vi "MapDeviceErrorToDescription.vi"(8 "error in":errorcluster {"code" format="%.0x"}, 11 "device error":u16 format="%.0x") -> (0 "error out":errorcluster {"code" format="%.0x"}, 3 "element":string)   [LabVIEW 2016]
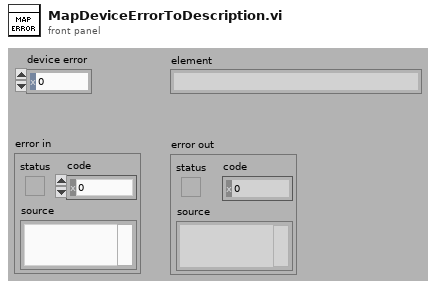
[diagram p1: front panel]
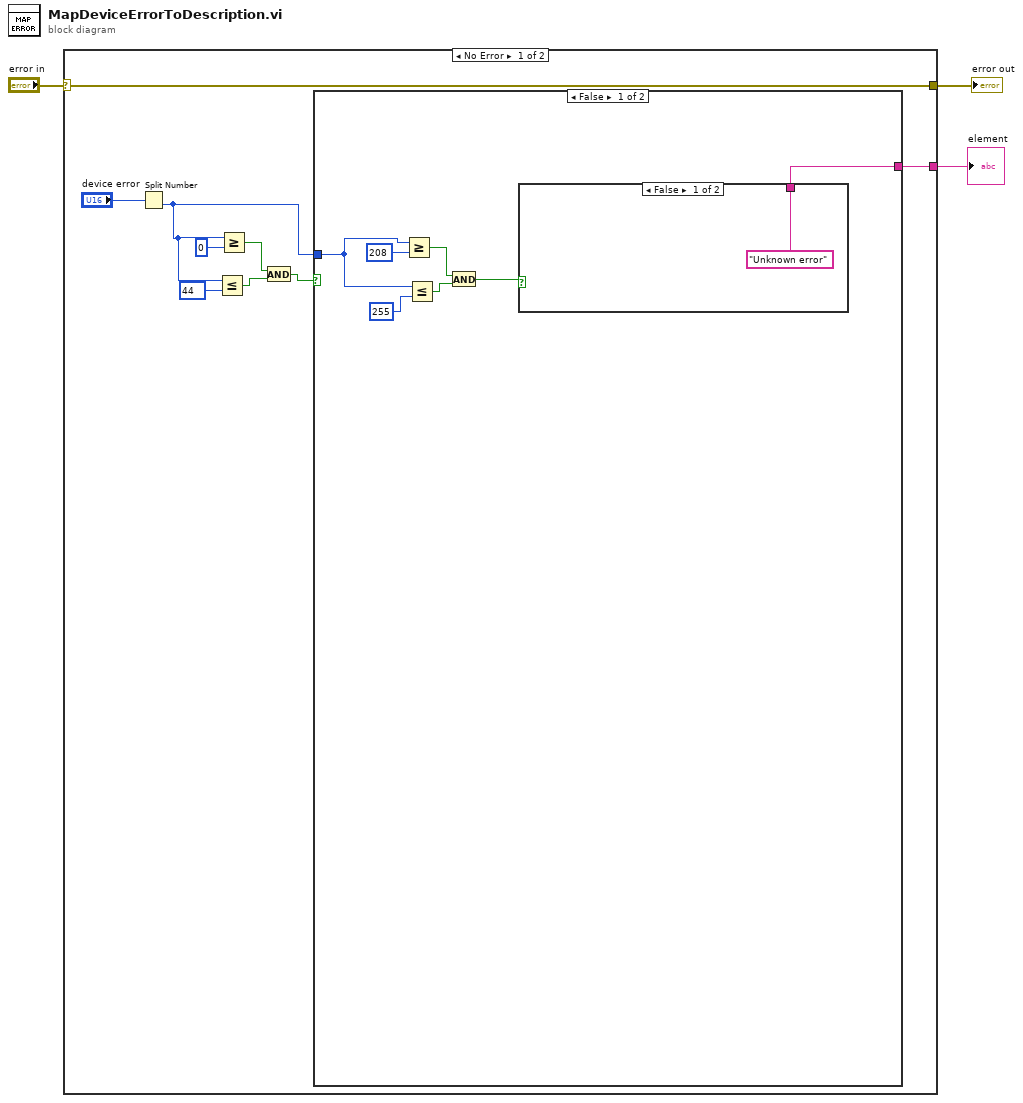
[diagram p0: block diagram]
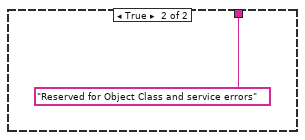
[diagram p2: hidden frame]
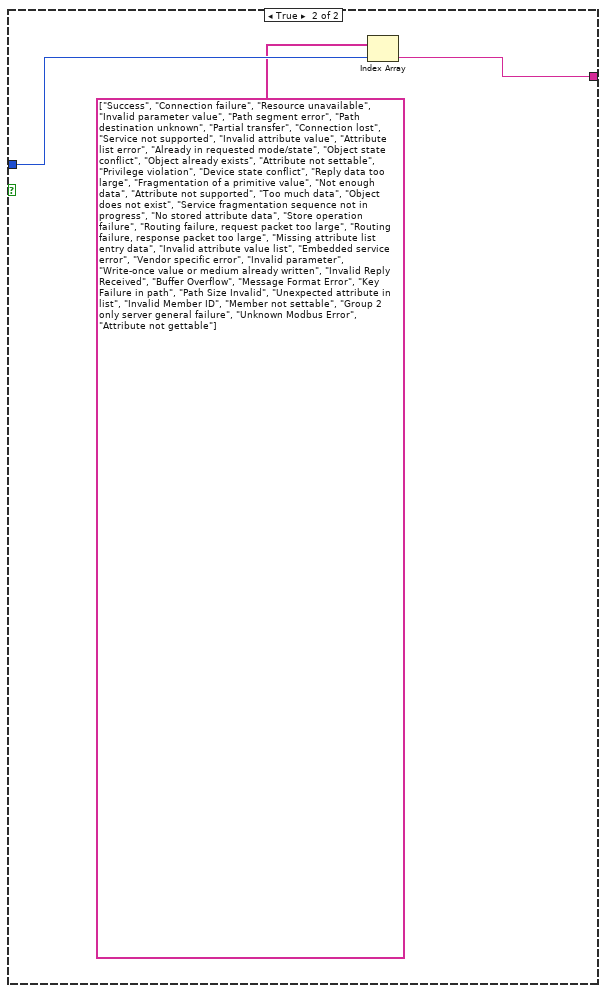
[diagram p3: hidden frame]
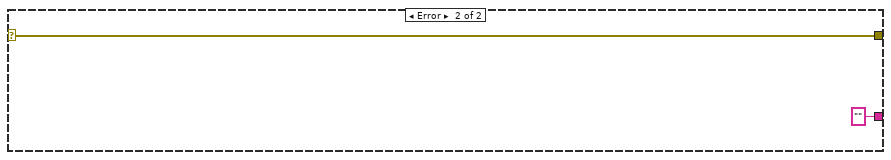
[diagram p4: hidden frame]
diagram:
  n1 = case shown="No Error" "error in" {
    selector: "error in" -> [w4 w26]
    tunnel: [w5 ""] -> w3
    tunnel: [w4 w26] -> w1
    frame No Error {
      n2 = Split Number(x="device error") -> (lo(x)=w6:u8)  [unwired: 1 out]
      n3 = Less Or Equal?(x=w6, y=u8 44) -> (x <= y?=w9:bool)
      n4 = Greater Or Equal?(x=w6, y=u8 0) -> (x >= y?=w10:bool)
      n5 = And(x=w10, y=w9) -> (x .and. y?=w7:bool)
      n6 = case shown="False" w7 {
        tunnel: w6 -> [w13 w24]
        tunnel: [w16 w22] -> w5
        frame False {
          n7 = Greater Or Equal?(x=w13, y=u8 208) -> (x >= y?=w18:bool)
          n8 = Less Or Equal?(x=w13, y=u8 255) -> (x <= y?=w15:bool)
          n9 = And(x=w18, y=w15) -> (x .and. y?=w17:bool)
          n10 = case shown="False" w17 {
            tunnel: ["Unknown error" "Reserved for Object Class and service errors"] -> w16
            frame False {
            }
            frame True {
            }
          }
        }
        frame True {
          n11 = Index Array(array=string[] ["Success", "Connection failure", "Resource unavailable", "Invalid parameter value", "Path segment error", "Path destination unknown", "Partial transfer", "Connection lost", "Service not supported", "Invalid attribute value", "Attribute list error", "Already in requested mode/state", "Object state conflict", "Object already exists", "Attribute not settable", "Privilege violation", "Device state conflict", "Reply data too large", "Fragmentation of a primitive value", "Not enough data", "Attribute not supported", "Too much data", "Object does not exist", "Service fragmentation sequence not in progress", "No stored attribute data", "Store operation failure", "Routing failure, request packet too large", "Routing failure, response packet too large", "Missing attribute list entry data", "Invalid attribute value list", "Embedded service error", "Vendor specific error", "Invalid parameter", "Write-once value or medium already written", "Invalid Reply Received", "Buffer Overflow", "Message Format Error", "Key Failure in path", "Path Size Invalid", "Unexpected attribute in list", "Invalid Member ID", "Member not settable", "Group 2 only server general failure", "Unknown Modbus Error", "Attribute not gettable"], index=w24) -> (element=w22:string)
        }
      }
    }
    frame Error {
    }
  }
  "element" <- w3
  "error out" <- w1
